vi "Update Custom Device Version in System Definition.vi"(8 "error in (no error)":errorcluster, 11 "Device Ref in":T1 format="%.0x") -> (0 "error out":errorcluster, 3 "Device Ref out":T1 format="%.0x")   [LabVIEW 2024, in "AIM ARINC 429 System Explorer.lvlib" / "Implementation.lvlib"]
uses:
  Implementation.lvlib
  <vilib>/NI VeriStand/Custom Device API/Custom Device Item Ref.ctl
  NationalInstruments.VeriStand.SystemDefinitionAPI
  <vilib>/NI VeriStand/Custom Device API/Custom Device API.lvlib
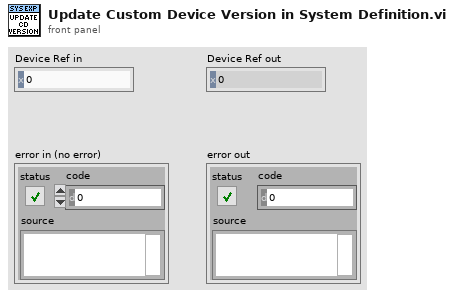
[diagram p1: front panel]
types:
  T1 = typedef "Custom Device API.lvlib/Custom Device Item Ref.ctl" = u64
  T2 = typedef "Custom Device API.lvlib/Custom Device Item Info.ctl" = cluster{"Name":string, "Is Channel":bool, "GUID":string, "Is Waveform":bool}
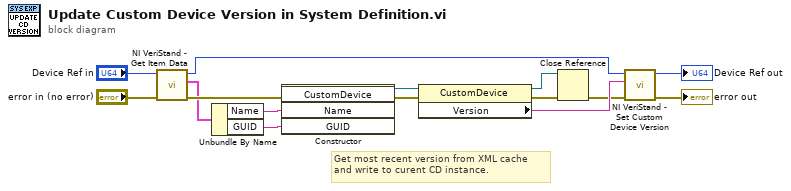
[diagram p0: block diagram]
diagram:
  # "Get most recent version from XML cache\nand write to curent CD instance."
  n1 = call <vilib>:"NI VeriStand - Get Item Data.vi"("error in (no error)"="error in (no error)", "Item Ref in"="Device Ref in") -> ("error out"=w4:errorcluster, "Item Info"=w1:T2, "Item Ref out"=w11:T1)  [unwired: 6 in, 1 out]
  n2 = Unbundle By Name(w1) -> ("Name"=w2:string, "GUID"=w3:string)
  n3 = constructor class="CustomDevice"(error in=w4, "Name"=w2, "GUID"=w3) -> (reference out=w5:refnum<k24>, error out=w6:errorcluster)  [unwired: 2 in, 3 out]
  n4 = property class="CustomDevice"(reference=w5, error in=w6) -> (reference out=w8:refnum<k24>, error out=w7:errorcluster, "Version"=w10:string)
  n5 = Close Reference(reference=w8, error in (no error)=w7) -> (error out=w9:errorcluster)
  n6 = call <vilib>:"NI VeriStand - Set Custom Device Version.vi"("error in (no error)"=w9, "Value"=w10, "Device Ref in"=w11) -> ("error out"=→"error out":errorcluster, "Device Ref out"=→"Device Ref out":T1)  [unwired: 7 in]
